vi "Run Action_Do.vi"(8 "error in (no error)":errorcluster, 10 "Project Builder in":refnum<class "Project Builder.lvclass">, 11 "Set Version from Git Tag":refnum<class "Set Version from Git Tag.lvclass">) -> (0 "error out":errorcluster, 1 "Success?":bool, 3 "Report Array":refnum<class "Report Data.lvclass">[](array[class]))   [LabVIEW 2020, in "ProjectBuilder.lvlib" / "Set Version from Git Tag.lvclass"]
uses:
  Set Version from Git Tag.lvclass
  C:/Current projects/WS/LV32.2020..ProjectBuilder/Class/Action/Project Action/Project Action.lvclass
  Data/Report Data/Report Data.lvclass
  Project Builder/Project Builder.lvclass
  Version Data/Version Data.lvclass
  C:/Current projects/WS/LV32.2020..ProjectBuilder/Class/Data/Report Data/Report Data.lvclass
  Action/Project Action/Project Action.lvclass/Project Action.ctl
  <vilib>/AppBuilder/AB_API_Simple/Build Specification Version.ctl
  Set Version from Git Tag.lvclass/Set Version from Git Tag.ctl
  Version Data/Version Data.lvclass/Version Data.ctl
  Action/Project Action/Project Action.lvclass
  ProjectBuilder.lvlib
  <vilib>/AppBuilder/AB_API_Simple/NI_App_Builder_API.lvlib
  C:/Current projects/WS/LV32.2020..ProjectBuilder/Interface/Action Interface/Action Interface.lvclass
  C:/Current projects/WS/LV32.2020..ProjectBuilder/Class/Set Version from Git Tag/Set Version from Git Tag.lvclass
  C:/Current projects/WS/LV32.2020..ProjectBuilder/Class/Set Version from Git Tag/Version Data/Version Data.lvclass
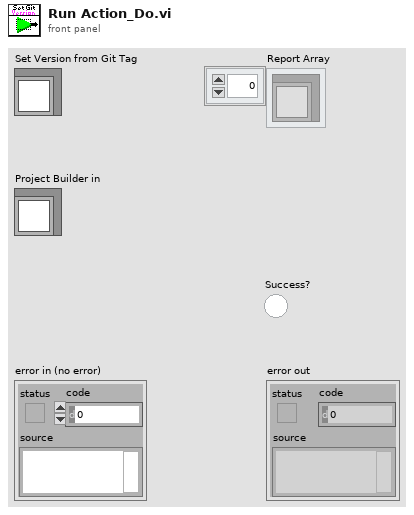
[diagram p1: front panel]
types:
  T1 = typedef "NI_App_Builder_API.lvlib/Build Specification Version.ctl" = cluster{"Major":u16, "Minor":u16, "Fix":u16, "Build":u16}
  T2 = cluster{"Build Specification Version[0]":i32, "Build Specification Version[1]":i32, "Build Specification Version[2]":i32, "Build Specification Version[3]":i32}
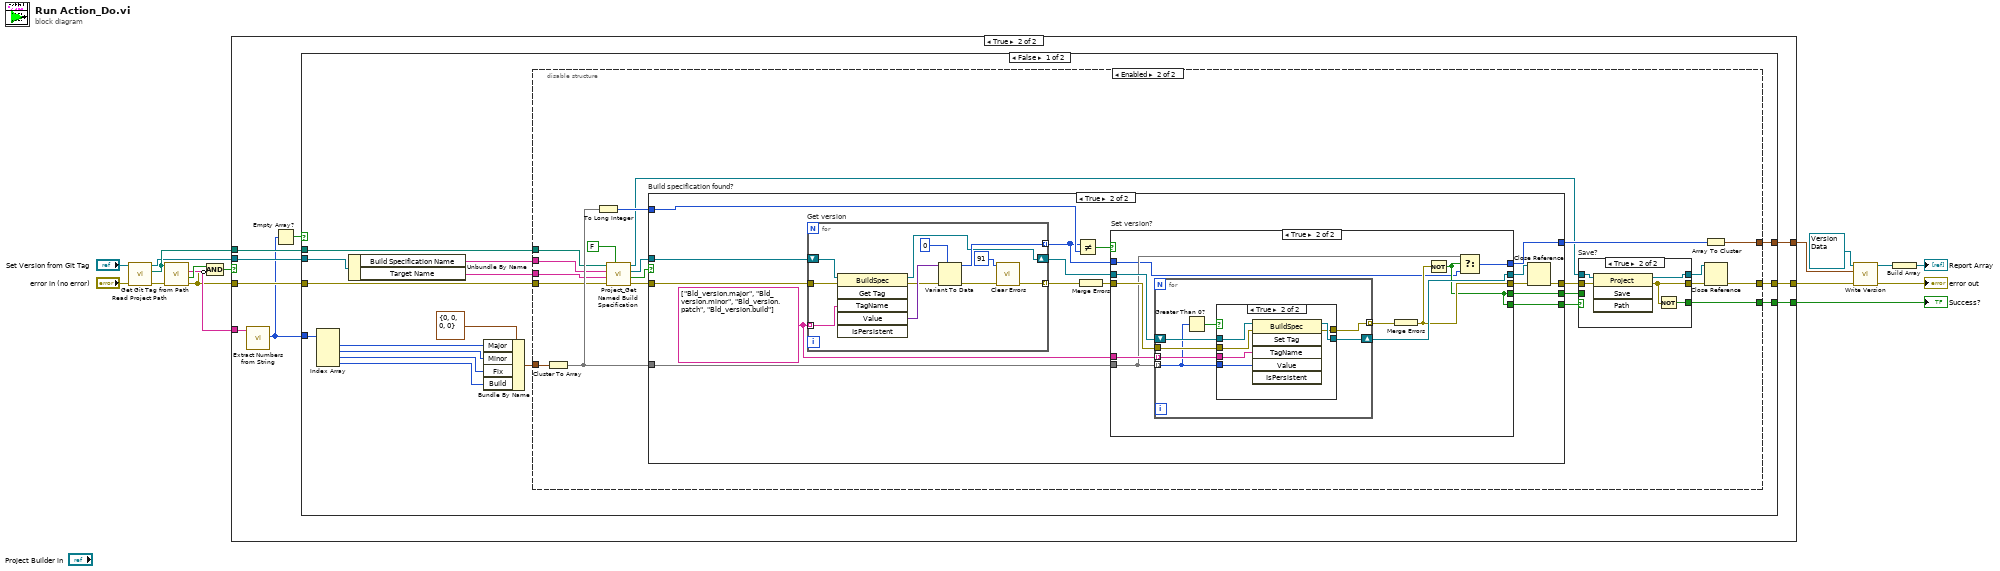
[diagram p0: block diagram]
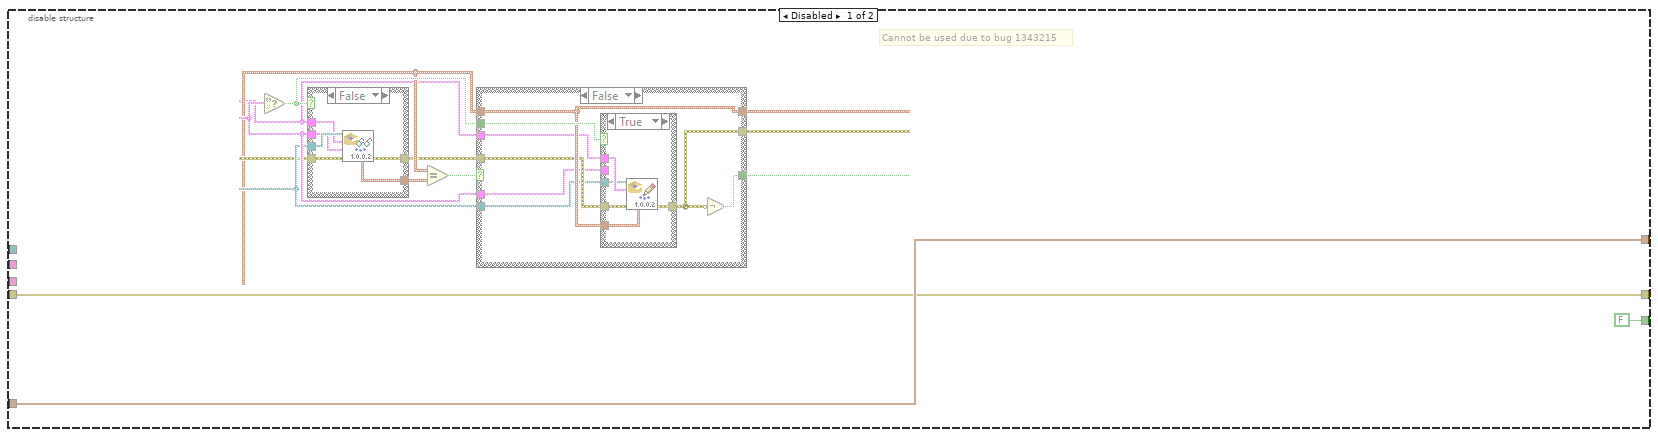
[diagram p3: hidden frame]
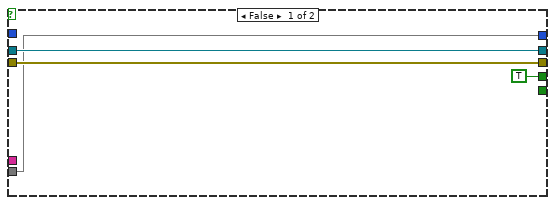
[diagram p5: hidden frame]
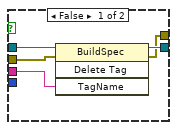
[diagram p6: hidden frame]
diagram:
  n1 = call "Read Project Path.vi"("error in (no error)"="error in (no error)", "Project Action in"="Set Version from Git Tag") -> ("error out"=w14:errorcluster, "Project Path"=w10:path, "Project Action out"=w8:refnum<class "Set Version from Git Tag.lvclass">)  [unwired: 7 in]
  n2 = call "Get Git Tag from Path.vi"("error in (no error)"=w14, "Path"=w10) -> ("error out"=w9:errorcluster, "Success?"=w13:bool, "Tag"=w11:string)  [unwired: 6 in, 1 out]
  n3 = Compound Arithmetic op=AND(w13, invert w9) -> (w12:bool)
  n4 = case shown="True" w12 {
    selector: w12 -> [w17 _]
    tunnel: w11 -> [_ w27]
    tunnel: w10 -> [_ w26]
    tunnel: [w18 w23] -> w7
    tunnel: w9 -> [w18 w24]
    tunnel: [w17 w22] -> w6
    tunnel: w8 -> [_ w25]
    tunnel: [_ w19] -> w1
    frame False {
    }
    frame True {
      n5 = call "Extract Numbers from String.vi"("String"=w27) -> ("Number Array"=w21:i32[])  [unwired: 9 in, 1 out]
      n6 = Empty Array?(array=w21) -> (empty?=w20:bool)
      n7 = case shown="False" w20 {
        tunnel: w26 -> [w29 _]
        tunnel: w25 -> [w37 _]
        tunnel: w24 -> [w30 w135]
        tunnel: [w28 w135] -> w23
        tunnel: [w36 _] -> w22
        tunnel: w21 -> [w35 _]
        tunnel: [w32 _] -> w19
        frame False {
          n8 = Index Array(array=w35) -> (element #1=w41:i32, element #2=w40:i32, element #3=w39:i32, element #4=w38:i32)  [unwired: 4 in]
          n9 = Unbundle By Name(w37) -> ("Build Specification Name"=w34:string, "Target Name"=w31:string)
          n10 = Bundle By Name(cluster=T1 {"Major"=0, "Minor"=0, "Fix"=0, "Build"=0} ("Build Specification Version"), "Major"=w41, "Minor"=w40, "Fix"=w39, "Build"=w38) -> (w33:T1)
          n11 = disable-structure shown="Enabled" {
            disable-tunnel: [FALSE w59] -> w36
            disable-tunnel: w34 -> [_ w54]
            disable-tunnel: w33 -> [w45 w64]
            disable-tunnel: [w45 w56] -> w32
            disable-tunnel: w31 -> [_ w46]
            disable-tunnel: w30 -> [w44 w55]
            disable-tunnel: w29 -> [_ w53]
            disable-tunnel: [w44 w60] -> w28
            frame Disabled {
              # "Cannot be used due to bug 1343215"
            }
            frame Enabled {
              n12 = Cluster To Array(cluster=w64) -> (array=w63:u16[])
              n13 = To Long Integer(number=w63) -> (32bit integer=w62:i32[])
              n14 = call "Project_Get Named Build Specification.vi"("Close project reference(T)"=FALSE, "error in(no error)"=w55, "Target Name(\"\"> My Computer)"=w46, "Build Specification Name"=w54, "Project Path"=w53) -> ("error out"=w49:errorcluster, "Success?"=w51:bool, "Build Spec reference"=w50:refnum<vi>, "Project reference (if not closed)"=w48:refnum<vi>)  [unwired: 3 in]
              n15 = case "Build specification found?" shown="True" w51 {
                tunnel: w49 -> [w67 w68]
                tunnel: [w67 w79] -> w47
                tunnel: w63 -> [_ w76]
                tunnel: w62 -> [_ w74]
                tunnel: [_ w73] -> w61
                tunnel: [_ w72] -> w58
                tunnel: [_ w70] -> w57
                tunnel: w50 -> [_ w69]
                frame False {
                }
                frame True {
                  w77 = string[] ["Bld_version.major", "Bld_version.minor", "Bld_version.patch", "Bld_version.build"]
                  n16 = for "Get version" {
                    tunnel: w77 -> [w125] mode=indexing
                    tunnel: [w122] -> w71 mode=indexing
                    shift-right: [w121] -> w78
                    shift-left: w69 -> [w126]
                    tunnel: [w117] -> w81 mode=indexing
                    tunnel: w68 -> [w118]
                    n17 = invoke class="BuildSpec" method="Get Tag"(reference=w126, error in=w118, "TagName"=w125) -> (reference out=w121:refnum<vi>, error out=w120:errorcluster, "Value"=w124:variant)  [unwired: 3 in, 3 out]
                    n18 = Variant To Data(error in=w120, type=0, Variant=w124) -> (data=w122:i32, error out=w119:errorcluster)
                    n19 = call <vilib>:"Clear Errors.vi"("error in (no error)"=w119, "specific error code to clear (0: all)"=91) -> ("error out"=w117:errorcluster)  [unwired: 4 in, 1 out]
                  }
                  n20 = Not Equal?(x=w71, y=w74) -> (x != y?=w75:bool)
                  n21 = Merge Errors(w81) -> (w82:errorcluster)
                  n22 = case "Set version?" shown="True" w75 {
                    tunnel: [w87 w97] -> w83
                    tunnel: w82 -> [w86 w96]
                    tunnel: [w86 w92] -> w80
                    tunnel: w78 -> [w87 w94]
                    tunnel: w77 -> [_ w93]
                    tunnel: w76 -> [w84 w90]
                    tunnel: [_ w91] -> w73
                    tunnel: [TRUE w91] -> w72
                    tunnel: w71 -> [_ w89]
                    tunnel: [w84 w88] -> w70
                    frame False {
                    }
                    frame True {
                      n23 = for {
                        tunnel: w93 -> [w103] mode=indexing
                        shift-right: [w102] -> w97
                        shift-left: w94 -> [w104]
                        tunnel: w90 -> [w99] mode=indexing
                        tunnel: [w101] -> w95 mode=indexing
                        tunnel: w96 -> [w100]
                        n24 = Greater Than 0?(x=w99) -> (x > 0?=w98:bool)
                        n25 = case shown="True" w98 {
                          tunnel: w104 -> [w109 w115]
                          tunnel: w103 -> [w108 w114]
                          tunnel: [w107 w113] -> w102
                          tunnel: [w105 w112] -> w101
                          tunnel: w100 -> [w106 w111]
                          tunnel: w99 -> [_ w110]
                          frame False {
                            n26 = invoke class="BuildSpec" method="Delete Tag"(reference=w109, error in=w106, "TagName"=w108) -> (reference out=w107:refnum<vi>, error out=w105:errorcluster)  [unwired: 1 in, 2 out]
                          }
                          frame True {
                            n27 = invoke class="BuildSpec" method="Set Tag"(reference=w115, error in=w111, "TagName"=w114, "Value"=w110) -> (reference out=w113:refnum<vi>, error out=w112:errorcluster)  [unwired: 2 in, 4 out]
                          }
                        }
                      }
                      n28 = Merge Errors(w95) -> (w92:errorcluster)
                      n29 = Not(x=w92) -> (.not. x?=w91:bool)
                      n30 = Select(t=w90, s=w91, f=w89) -> (s? t:f=w88:i32[])
                    }
                  }
                  n31 = Close Reference(reference=w83, error in (no error)=w80) -> (error out=w79:errorcluster)
                }
              }
              n32 = case "Save?" shown="True" w61 {
                tunnel: [w128 w130] -> w66
                tunnel: [w129 w134] -> w65
                tunnel: w48 -> [w129 w133]
                tunnel: w47 -> [w128 w132]
                tunnel: [w127 w131] -> w59
                tunnel: w58 -> [w127 _]
                frame False {
                }
                frame True {
                  n33 = invoke class="Project" method="Save"(reference=w133, error in=w132) -> (reference out=w134:refnum<vi>, error out=w130:errorcluster)  [unwired: 2 in, 2 out]
                  n34 = Not(x=w130) -> (.not. x?=w131:bool)
                }
              }
              n35 = Array To Cluster(array=w57) -> (cluster=w56:T2)
              n36 = Close Reference(reference=w65, error in (no error)=w66) -> (error out=w60:errorcluster)
            }
          }
        }
        frame True {
        }
      }
    }
  }
  "Success?" <- w6
  n37 = call "Write Version.vi"("error in (no error)"=w7, "Build Specification Version"=w1, "Version Data in"=refnum<class "Version Data.lvclass"> refnum ("ProjectBuilder.lvlib:Version Data.lvclass")) -> ("error out"=→"error out":errorcluster, "Version Data out"=w2:refnum<class "Version Data.lvclass">)  [unwired: 7 in]
  n38 = Build Array(w2) -> (→"Report Array":refnum<class "Version Data.lvclass">[])
